vi "Return Device Activate Status.vi"(4 "error string":string, 6 "Status":T1, 8 "error in (no error)":errorcluster, 10 "IED Name":string, 11 "SCADA in":refnum<class "SCADA.lvclass">) -> (0 "error out":errorcluster, 3 "SCADA out":refnum<class "SCADA.lvclass">)   [LabVIEW 2015, in "SCADA Core.lvlib" / "SCADA.lvclass"]
uses:
  SCADA.lvclass
  SCADA Abstract Messages/Device Action Status Msg/Device Action Status.ctl
  <vilib>/ActorFramework/Actor/Actor.lvclass/Actor.ctl
  SCADA.lvclass/SCADA.ctl
  <vilib>/ActorFramework/Actor/Actor.lvclass
  SCADA Abstract Messages/Device Action Status Msg/Device Action Status Msg.lvclass
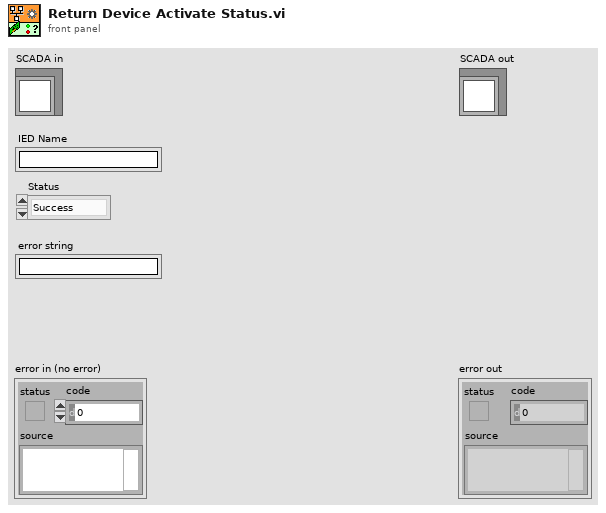
[diagram p1: front panel]
types:
  T1 = typedef "SCADA Core.lvlib/Device Action Status Msg.lvclass/Device Action Status.ctl" = enum16{"Success", "Failure"}
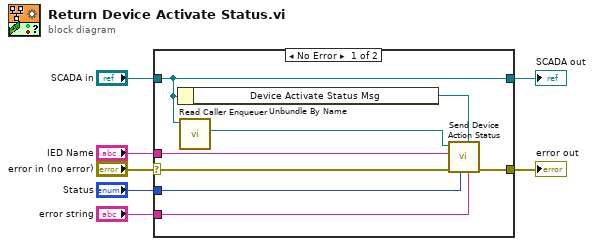
[diagram p0: block diagram]
diagram:
  n1 = case shown="No Error" "error in (no error)" {
    selector: "error in (no error)" -> [w11 w17]
    tunnel: [w8 w17] -> w6
    tunnel: [w15 w16] -> w4
    tunnel: "SCADA in" -> [w15 w16]
    tunnel: "IED Name" -> [w14 _]
    tunnel: "Status" -> [w10 _]
    tunnel: "error string" -> [w9 _]
    frame No Error {
      n2 = Unbundle By Name(w15) -> ("Device Activate Status Msg"=w13:refnum<class "Device Action Status Msg.lvclass">)
      n3 = call <vilib>:"Read Caller Enqueuer.vi"("Actor"=w15) -> ("Caller Enqueuer"=w12:refnum<class "Message Enqueuer.lvclass">)  [unwired: 10 in]
      n4 = call "Send Device Action Status.vi"("error string"=w9, "Island Control Status Msg"=w13, "Status"=w10, "error in (no error)"=w11, "IED Name"=w14, "Message Enqueuer in"=w12) -> ("error out"=w8:errorcluster)  [unwired: 4 in, 1 out]
    }
    frame Error {
    }
  }
  "error out" <- w6
  "SCADA out" <- w4
